vi "SetDefaultStage.vi"(8 "error in (no error)":errorcluster, 10 "DefaultStageEnqueuer":refnum<class "Message Enqueuer.lvclass">, 11 "Microscope in":refnum<class "Microscope.lvclass">) -> (0 "error out":errorcluster, 3 "Microscope out":refnum<class "Microscope.lvclass">)   [LabVIEW 2020, in "Microscope.lvlib" / "Microscope.lvclass"]
uses:
  Microscope.lvclass
  C:/Program Files/National Instruments/LabVIEW 2020/vi.lib/ActorFramework/Actor/Actor.lvclass
  <vilib>/ActorFramework/Message Enqueuer/Message Enqueuer.lvclass
  Microscope.lvclass/Microscope.ctl
  <vilib>/ActorFramework/Actor/Actor.lvclass/Actor.ctl
  <vilib>/ActorFramework/Message Enqueuer/Message Enqueuer.lvclass/Message Enqueuer.ctl
  Interface/DataGenerator Messages/AddDataListener Msg/AddDataListener Msg.lvclass/AddDataListener Msg.ctl
  <vilib>/ActorFramework/Message Enqueuer/Init from Existing Queue.vi
  <vilib>/ActorFramework/Message Enqueuer/Enqueue.vi
  Interface/DataGenerator Messages/AddDataListener Msg/AddDataListener Msg.lvclass
  C:/Program Files/National Instruments/LabVIEW 2020/vi.lib/ActorFramework/Message/Message.lvclass
  <vilib>/ActorFramework/Message Priority Queue/Priority Enqueue.vi
  <vilib>/ActorFramework/Actor/Actor.lvclass
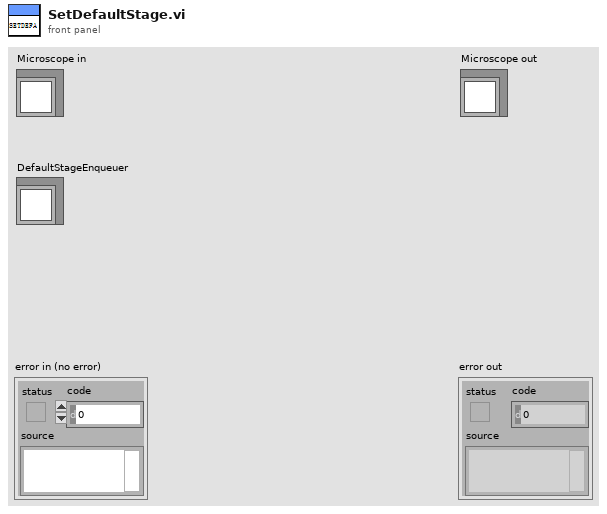
[diagram p1: front panel]
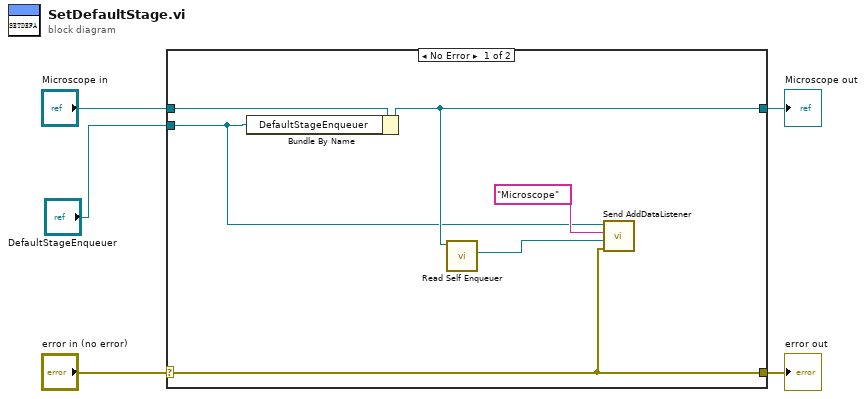
[diagram p0: block diagram]
diagram:
  n1 = case shown="No Error" "error in (no error)" {
    selector: "error in (no error)" -> [w6 w13]
    tunnel: [w6 w13] -> w4
    tunnel: [w8 w12] -> w2
    tunnel: "Microscope in" -> [w11 w12]
    tunnel: "DefaultStageEnqueuer" -> [w7 _]
    frame No Error {
      n2 = Bundle By Name(cluster=w11, "DefaultStageEnqueuer"=w7) -> (w8:refnum<class "Microscope.lvclass">)
      n3 = call <vilib>:"Read Self Enqueuer.vi"("Actor"=w8) -> ("Self Enqueuer"=w10:refnum<class "Message Enqueuer.lvclass">)  [unwired: 10 in]
      n4 = call "Send AddDataListener.vi"("error in (no error)"=w6, "Listener In"=w10, "Label"="Microscope", "Message Enqueuer"=w7) -> ()  [unwired: 6 in, 2 out]
    }
    frame Error {
    }
  }
  "error out" <- w4
  "Microscope out" <- w2
